vi "Read_From_Port.vi"() -> ()   [LabVIEW 2015]
uses:
  <vilib>/Utility/error.llb/DialogType.ctl
panel:
  in  "data to MATLAB":string
  out "incoming bytes":string
  in  "stop":bool
  out "Data From MATLAB":string
  in  "Port":u16=2057 caption="Port to Connect" min=1025 step=1
  in  "IP-Addresse":string="localhost" caption="IP-Adresse"
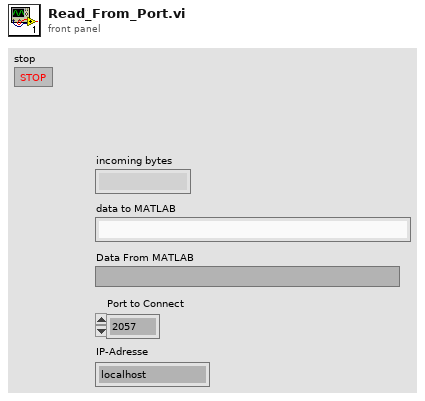
[diagram p1: front panel]
types:
  T1 = enum16{"Standard", "Buffered", "CRLF", "Immediate"}
  T2 = typedef "DialogType.ctl" = u16
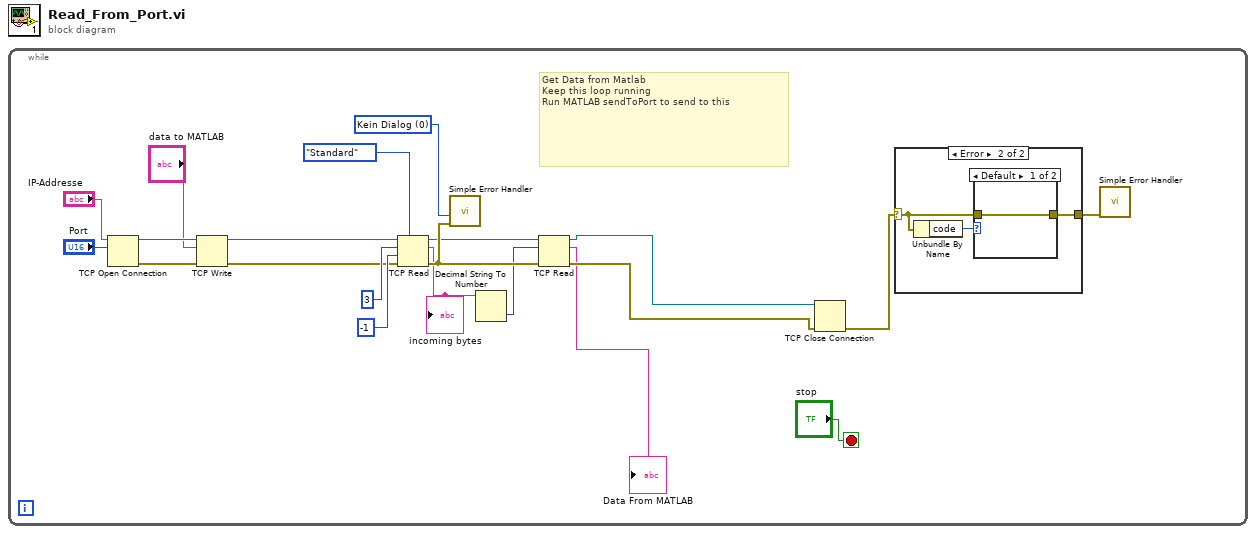
[diagram p0: block diagram]
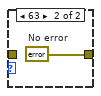
[diagram p3: hidden frame]
diagram:
  n1 = while {
    stop <- "stop" stop-if-true
    w20 = T2 0 items=["Kein Dialog", "OK-Meldung", "Dialog zum Fortsetzen oder Anhalten", "OK-Meldung + Warnungen", "Weiter/Stopp + Warnung"] ("type of dialog (OK msg:1)")
    # "Get Data from Matlab\nKeep this loop running\nRun MATLAB sendToPort to send to this"
    n2 = TCP Open Connection(address="IP-Addresse", remote port or service name="Port") -> (connection ID=w3:refnum<k5>, error out=w5:errorcluster)  [unwired: 3 in]
    n3 = TCP Write(connection ID=w3, data in="data to MATLAB", error in (no error)=w5) -> (connection ID out=w2:refnum<k5>, error out=w4:errorcluster)  [unwired: 1 in, 1 out]
    n4 = TCP Read(connection ID=w2, bytes to read=3 ("Zu lesende Bytes"), error in (no error)=w4, 7:T1."Standard" ("Modus (Standard)"), 9:-1 ("Timeout in ms (25000)")) -> (connection ID out=w13:refnum<k5>, data out=w9:string, error out=w14:errorcluster)
    "incoming bytes" <- w9
    n5 = call <vilib>:"Simple Error Handler.vi"("type of dialog (OK msg:1)"=w20, "error in (no error)"=w14) -> ()  [unwired: 3 in, 5 out]
    n6 = Decimal String To Number(string=w9) -> (number=w8:i32)  [unwired: 2 in, 1 out]
    n7 = TCP Read(connection ID=w13, bytes to read=w8, error in (no error)=w14) -> (connection ID out=w11:refnum<k5>, data out=→"Data From MATLAB":string, error out=w12:errorcluster)  [unwired: 2 in]
    n8 = TCP Close Connection(connection ID=w11, error in (no error)=w12) -> (error out=w7:errorcluster)  [unwired: 1 in, 1 out]
    n9 = case shown="Error" w7 {
      selector: w7 -> [w22 w24]
      tunnel: [w22 w23] -> w15
      frame No Error {
      }
      frame Error {
        n10 = Unbundle By Name(w24) -> ("code"=w25:i32)
        n11 = case shown="Default" w25 {
          tunnel: w24 -> [w26 _]
          tunnel: [w26 w27] -> w23
          frame Default {
          }
          frame 63 {
            w27 = errorcluster {"status"=FALSE, "code"=0, "source"=""}  # No error
          }
        }
      }
    }
    n12 = call <vilib>:"Simple Error Handler.vi"("error in (no error)"=w15) -> ()  [unwired: 4 in, 5 out]
  }
